vi "5302GetTCVISA.vi"(8 "error in (no error)":errorcluster, 11 "VISA session (for class)":refnum<visa-resource-name>) -> (0 "error out":errorcluster, 1 "data string":string, 2 "Time Constant":dbl format="%.4e", 3 "VISA session":refnum<visa-resource-name>)   [LabVIEW 2015]
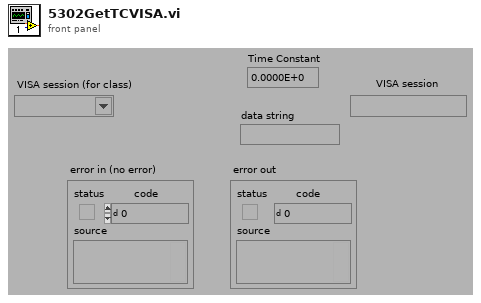
[diagram p1: front panel]
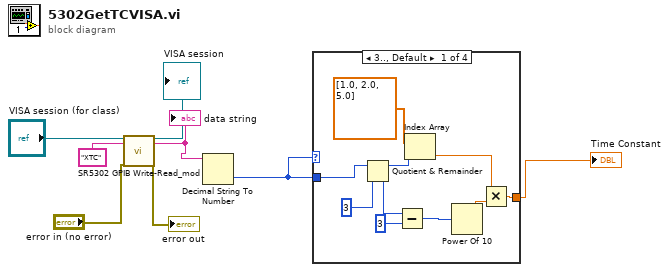
[diagram p0: block diagram]
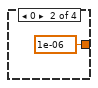
[diagram p2: hidden frame]
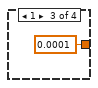
[diagram p3: hidden frame]
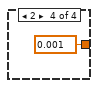
[diagram p4: hidden frame]
diagram:
  n1 = call "SR5302 GPIB Write-Read_mod.vi"("VISA session (for class)"="VISA session (for class)", "Write Command String"="XTC" ("data string"), "error in (no error)"="error in (no error)") -> ("VISA session"=→"VISA session":refnum<visa-resource-name>, "Response 1"=w3:string, "error out"=→"error out":errorcluster)  [unwired: 5 in, 9 out]
  "data string" <- w3
  n2 = Decimal String To Number(string=w3) -> (number=w4:i32)  [unwired: 2 in, 1 out]
  n3 = case shown="3.., Default" w4 {
    tunnel: [w16 1e-06 0.0001 0.001] -> w5
    tunnel: w4 -> [w15 _ _ _]
    frame 3.., Default {
      n4 = Quotient & Remainder(x=w15, y=3) -> (x-y*floor(x/y)=w11:i32, floor(x/y)=w13:i32)
      n5 = Subtract(x=w13, y=3) -> (x-y=w14:i32)
      n6 = Index Array(array=dbl[] [1.0, 2.0, 5.0] ("Input Array"), index=w11) -> (element=w9:dbl)
      n7 = Power Of 10(x=w14) -> (10^x=w17:dbl)
      n8 = Multiply(x=w9, y=w17) -> (x*y=w16:dbl)
    }
    frame 0 {
    }
    frame 1 {
    }
    frame 2 {
    }
  }
  "Time Constant" <- w5
